vi "Demo_GenSine.vi"() -> ()   [LabVIEW 2020]
panel:
  in  "Stop":bool
  in  "Generate Sine":bool
  out "Constant Signal":dbl[](graph)
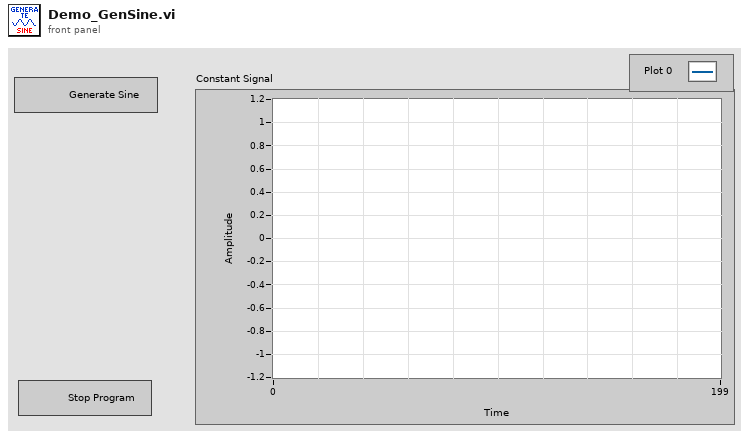
[diagram p1: front panel]
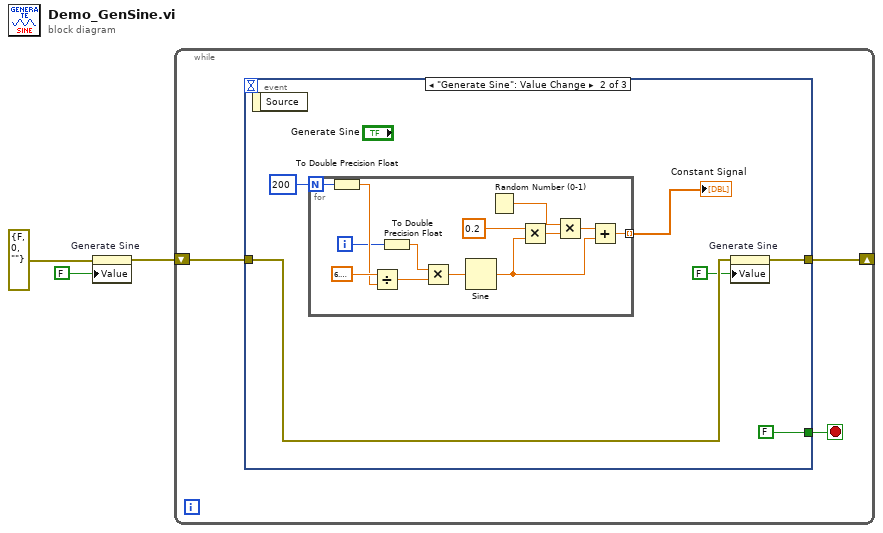
[diagram p0: block diagram]
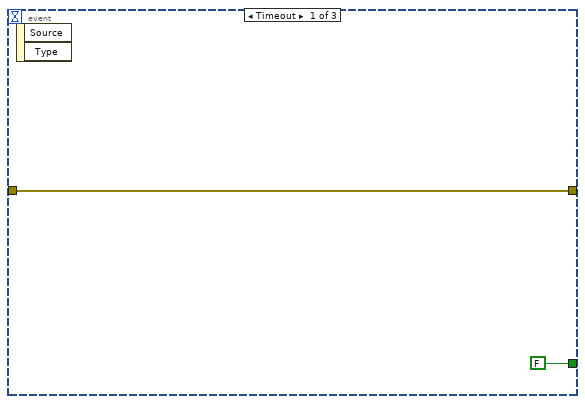
[diagram p2: hidden frame]
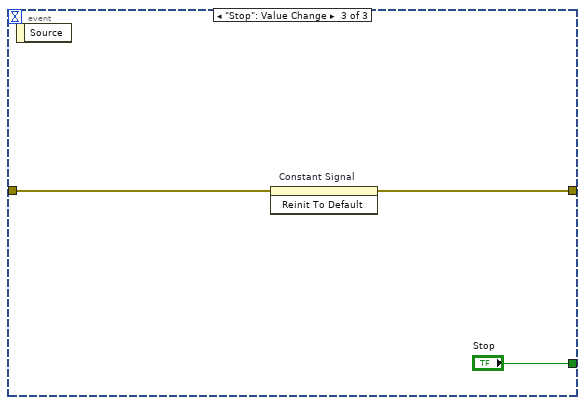
[diagram p3: hidden frame]
diagram:
  n1 = property on="Generate Sine" class="Bool (strict)"(error in=errorcluster {"status"=FALSE, "code"=0, "source"=""} ("error in (no error)"), "Value"=FALSE ("Generate Sine")) -> (error out=w2:errorcluster)  [unwired: 1 in, 1 out]
  n2 = while {
    shift-right: [w4] -> _
    shift-left: w2 -> [w5]
    stop <- w6 stop-if-true
    n3 = event shown="[1] \"Generate Sine\": Value Change" {
      selector: _ -> [_ _ _]
      dyn-events: _ -> [_ _ _]
      timeout: _ -> [_ _ _]
      tunnel: [FALSE ("Stop") FALSE ("Stop") "Stop"] -> w6
      tunnel: w5 -> [w7 w11 w29]
      tunnel: [w7 w12 w28] -> w4
      event Timeout {
        n4 = event-data() -> ()  [unwired: 1 in, 2 out]
      }
      event "Generate Sine": Value Change {
        n5 = event-data() -> ()  [unwired: 1 in, 1 out]
        n6 = for {
          N: 200 -> [w26]
          tunnel: [w15] -> w9 mode=indexing
          i -> [w23]
          n7 = To Double Precision Float(number=w26) -> (double precision float=w25:dbl)
          n8 = Divide(x=6.283185307179586, y=w25) -> (x/y=w24:dbl)
          n9 = To Double Precision Float(number=w23) -> (double precision float=w22:dbl)
          n10 = Multiply(x=w22, y=w24) -> (x*y=w21:dbl)
          n11 = Sine(x=w21) -> (sin(x)=w16:dbl)
          n12 = Random Number (0-1)() -> (number: 0 to 1=w19:dbl)
          n13 = Multiply(x=0.2, y=w16) -> (x*y=w18:dbl)
          n14 = Multiply(x=w19, y=w18) -> (x*y=w17:dbl)
          n15 = Add(x=w17, y=w16) -> (x+y=w15:dbl)
        }
        "Constant Signal" <- w9
        n16 = property on="Generate Sine" class="Bool (strict)"(error in=w11, "Value"=FALSE ("Generate Sine")) -> (error out=w12:errorcluster)  [unwired: 1 in, 1 out]
      }
      event "Stop": Value Change {
        n17 = event-data() -> ()  [unwired: 1 in, 1 out]
        n18 = invoke on="Constant Signal" class="WFGraph (strict)" method="Reinit To Default"(error in=w29) -> (error out=w28:errorcluster)  [unwired: 2 in, 2 out]
      }
    }
  }
